vi "addFailure.vi"(7 "execution time (sec)":dbl, 8 "error in (no error)":errorcluster, 9 "test error":errorcluster, 10 "test":refnum<class>, 11 "TestTestResult in":refnum<class "_TextTestResult.JUnitXML.lvclass">) -> (0 "error out":errorcluster, 3 "TestTestResult out":refnum<class "_TextTestResult.JUnitXML.lvclass">)   [LabVIEW 2018, in "_TextTestResult.JUnitXML.lvclass"]
uses:
  _TextTestResult.JUnitXML.lvclass
  <vilib>/addons/_JKI Toolkits/VI Tester/TestResult.llb/resultStatus--enum.ctl
  <vilib>/addons/_JKI Toolkits/VI Tester/_TextTestResult.llb/_TextTestResult.lvclass
  <vilib>/addons/_JKI Toolkits/VI Tester/TestResult.llb/TestResult.lvclass
panel:
  # "JKI VI Tester for LabVIEW\nhttp://jkisoft.com/vi-tester\nCopyright (C) 2007-2009, JKI <info@jkisoft.com>\nALL RIGHTS RESERVED"
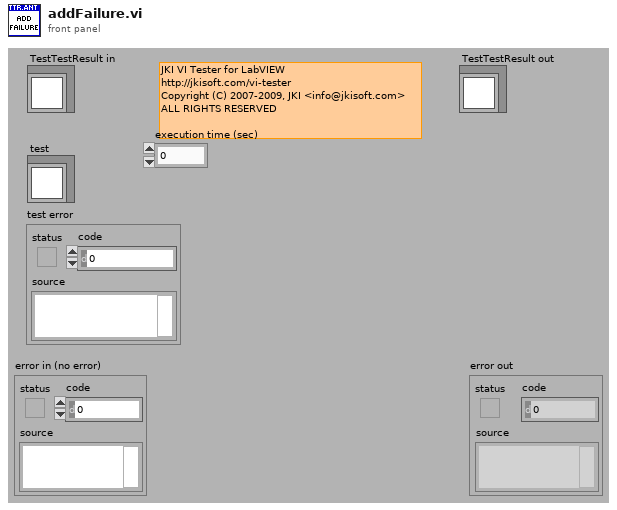
[diagram p1: front panel]
types:
  T1 = typedef "TestResult.lvclass/resultStatus--enum.ctl" = enum16{"testPass", "testFailure", "testError", "testSkipped"}
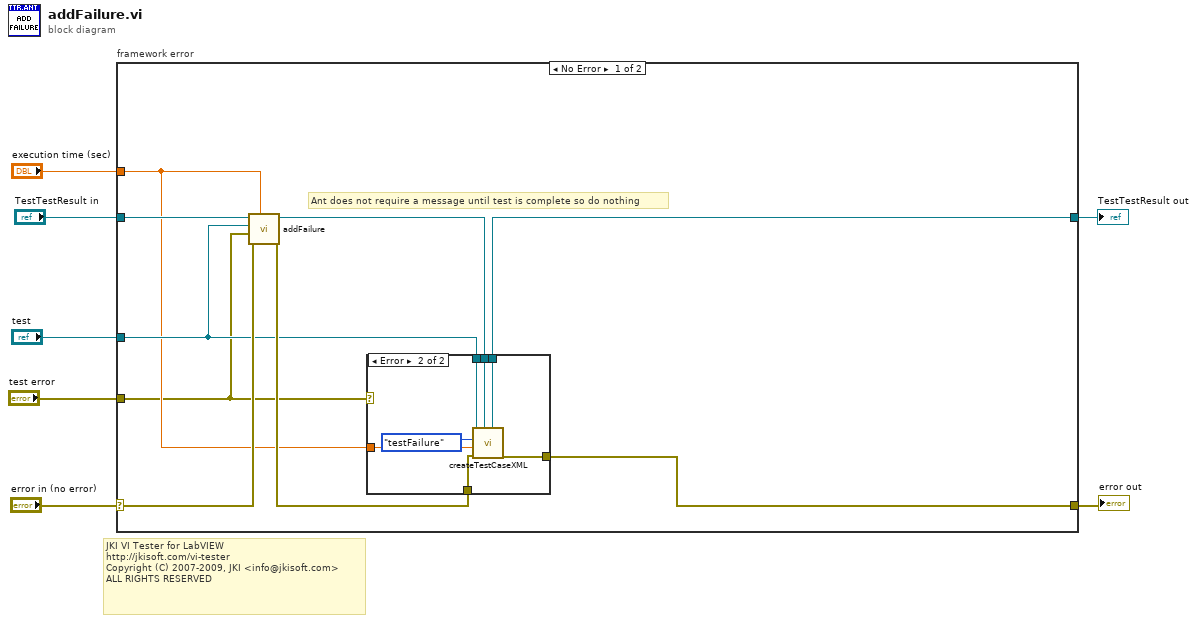
[diagram p0: block diagram]
diagram:
  # "JKI VI Tester for LabVIEW\nhttp://jkisoft.com/vi-tester\nCopyright (C) 2007-2009, JKI <info@jkisoft.com>\nALL RIGHTS RESERVED"
  n1 = case "framework error" shown="No Error" "error in (no error)" {
    selector: "error in (no error)" -> [w15 w27]
    tunnel: [w11 w27] -> w6
    tunnel: [w8 w26] -> w4
    tunnel: "TestTestResult in" -> [w16 w26]
    tunnel: "test" -> [w13 _]
    tunnel: "test error" -> [w10 _]
    tunnel: "execution time (sec)" -> [w12 _]
    frame No Error {
      # "Ant does not require a message until test is complete so do nothing"
      n2 = call-parent "addFailure.vi"("execution time (sec)"=w12, "error in (no error)"=w15, "test error"=w10, "test"=w13, "TestTestResult in"=w16) -> ("error out"=w14:errorcluster, "TestTestResult out"=w9:refnum<class "_TextTestResult.JUnitXML.lvclass">)  [unwired: 5 in]
      n3 = case shown="Error" w10 {
        tunnel: w14 -> [w18 w24]
        tunnel: w13 -> [_ w23]
        tunnel: w12 -> [_ w22]
        tunnel: w9 -> [w17 w21]
        tunnel: [w18 w20] -> w11
        tunnel: [w17 w19] -> w8
        frame No Error {
        }
        frame Error {
          n4 = call "createTestCaseXML.vi"("TestTestResult.Ant"=w21, "error in (no error)"=w24, "execution time (sec)"=w22, "resultStatus"=resultStatus--enum."testFailure", "Test Out"=w23) -> ("error out"=w20:errorcluster, "TestTestResult.Ant Out"=w19:refnum<class "_TextTestResult.JUnitXML.lvclass">)  [unwired: 5 in]
        }
      }
    }
    frame Error {
    }
  }
  "error out" <- w6
  "TestTestResult out" <- w4
